vi "Write SP.vi"(8 "error in (no error)":errorcluster, 10 "SP":dbl, 11 "Change Setpoint MSG in":refnum<class "Change Setpoint MSG.lvclass">) -> (0 "error out":errorcluster, 3 "Change Setpoint MSG out":refnum<class "Change Setpoint MSG.lvclass">)   [LabVIEW 2014, in "Alicat Lib.lvlib" / "Change Setpoint MSG.lvclass"]
uses:
  Change Setpoint MSG.lvclass
  Change Setpoint MSG.lvclass/Change Setpoint MSG.ctl
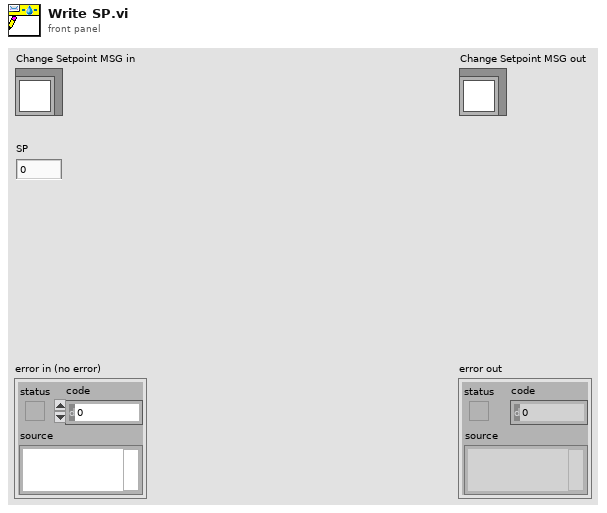
[diagram p1: front panel]
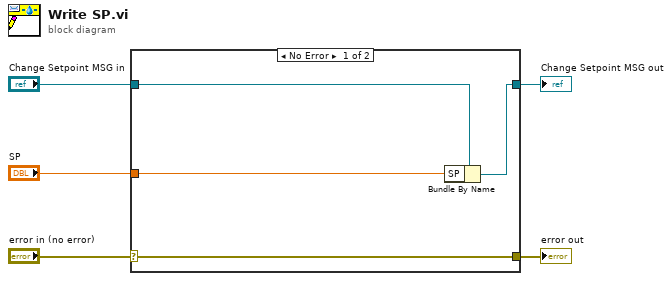
[diagram p0: block diagram]
diagram:
  n1 = case shown="No Error" "error in (no error)" {
    selector: "error in (no error)" -> [w9 w10]
    tunnel: [w9 w10] -> w4
    tunnel: [w7 w11] -> w2
    tunnel: "Change Setpoint MSG in" -> [w8 w11]
    tunnel: "SP" -> [w6 _]
    frame No Error {
      n2 = Bundle By Name(cluster=w8, "SP"=w6) -> (w7:refnum<class "Change Setpoint MSG.lvclass">)
    }
    frame Error {
    }
  }
  "error out" <- w4
  "Change Setpoint MSG out" <- w2
